vi "Aircraft 6 RC Override Values.vi"(7 "Method":enum16{"Get", "Set"}(ring), 11 "Auto Override Values":T1) -> (3 "Auto Override Values Out":T1)   [LabVIEW 2014]
uses:
  Controls/RC Override.ctl
  Controls/Aircraft Mode.ctl
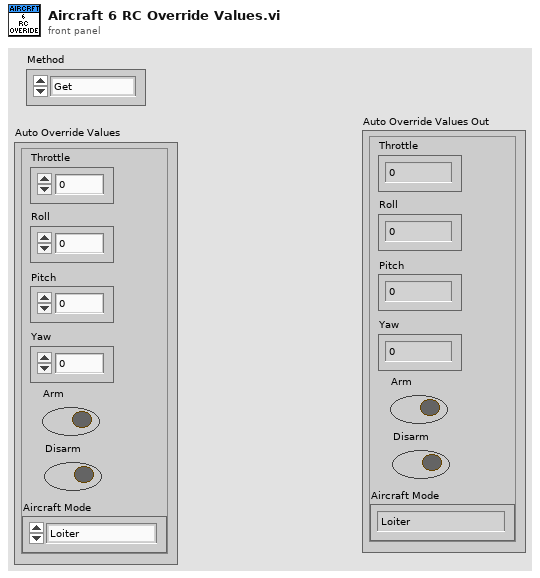
[diagram p1: front panel]
types:
  T1 = typedef "RC Override.ctl" = cluster{"Throttle":u16, "Roll":u16, "Pitch":u16, "Yaw":u16, "Arm":bool, "Disarm":bool, "Aircraft Mode":T2}
  T2 = typedef "Aircraft Mode.ctl" = enum16{"Loiter", "Stabalise", "Failsafe", "Emergency Stop"}
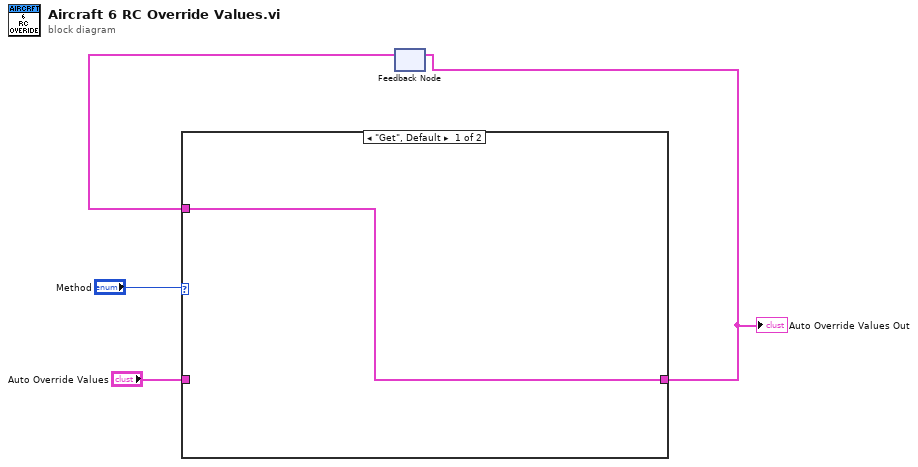
[diagram p0: block diagram]
diagram:
  n1 = feedback #1() -> (w1:T1)  [unwired: 1 in]
  n2 = case shown="\"Get\", Default" "Method" {
    tunnel: "Auto Override Values" -> [_ w6]
    tunnel: [w5 w6] -> w2
    tunnel: w1 -> [w5 _]
    frame "Get", Default {
    }
    frame "Set" {
    }
  }
  "Auto Override Values Out" <- w2
  n3 = feedback-in #1(w2) -> ()
